vi "MCL Move Z Center.vi"(8 "error in (no error)":errorcluster, 9 "handle":i32, 10 "actual":dbl, 11 "position":dbl) -> (0 "error out":errorcluster, 2 "actual out":dbl, 3 "function return":i32)   [LabVIEW 2014, in "Madlib.lvlib"]
doc: "MADLIB_API int MCL_MoveZCenter(double position, double *actual, int handle);"
uses:
  <userlib>/Lambda2/lib/Madlib/Madlib.lvlib
  <userlib>/Lambda2/lib/Madlib/Madlib.dll
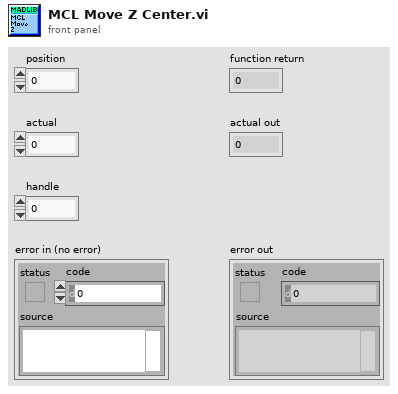
[diagram p1: front panel]
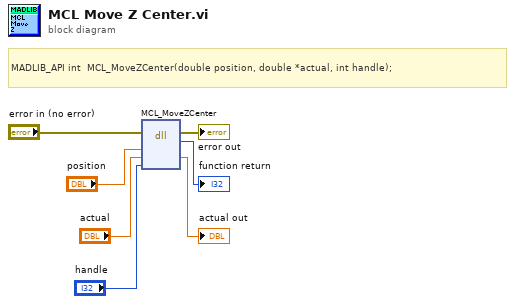
[diagram p0: block diagram]
diagram:
  # "MADLIB_API\tint\t\tMCL_MoveZCenter(double position, double *actual, int handle);"
  n1 = dll-call lib="C:/Program Files (x86)/National Instruments/LabVIEW 2014/user.lib/Lambda2/lib/Madlib/Madlib.*" fn="MCL_MoveZCenter"(error in="error in (no error)", "position"="position", "actual"="actual", "handle"="handle") -> (error out=→"error out":errorcluster, →"function return":i32, "actual"=→"actual out":dbl)  [unwired: 4 in, 1 out]
